vi "User_Palette.vi"(10 "Color":u32(colorbox), 11 "Palette Number (gray)":T1(ring)) -> (3 "Color Palette":cluster{"Red":u8, "Green":u8, "Blue":u8}[](array[cluster]))   [LabVIEW 2013]
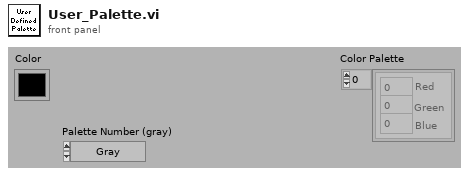
[diagram p1: front panel]
types:
  T1 = enum32{"Gray", "Binary", "Gradient", "Rainbow", "Temperature", "User Defined"}
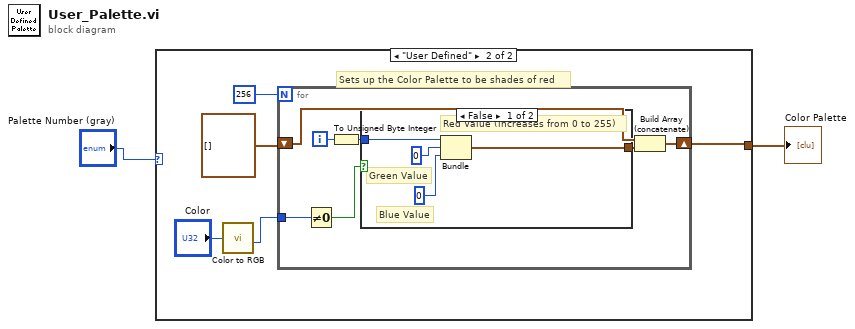
[diagram p0: block diagram]
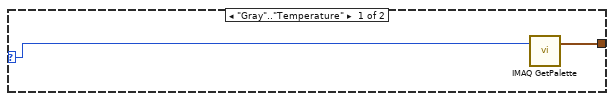
[diagram p2: hidden frame]
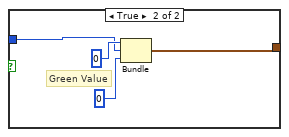
[diagram p3: hidden frame]
diagram:
  n1 = case shown="\"User Defined\"" "Palette Number (gray)" {
    selector: "Palette Number (gray)" -> [w3 _]
    tunnel: [w4 w7] -> w2
    frame "Gray".."Temperature" {
      n2 = call "IMAQ GetPalette"("Palette Number (gray)"=w3) -> ("Color Palette"=w4:cluster{"Red":u8, "Green":u8, "Blue":u8}[])  [unwired: 4 in, 1 out]
    }
    frame "User Defined" {
      # "Sets up the Color Palette to be shades of red"
      n3 = call <vilib>:"Color to RGB.vi"("Color"="Color") -> ("G"=w5:u8)  [unwired: 3 out]
      n4 = for {
        N: 256 -> [_]
        shift-right: [w14] -> w7
        shift-left: cluster{u8, "G":u8, u8}[] [] -> [w15]
        tunnel: w5 -> [w10]
        i -> [w13]
        n5 = Not Equal To 0?(x=w10) -> (x != 0?=w11:bool)
        n6 = To Unsigned Byte Integer(number=w13) -> (unsigned 8bit integer=w12:u8)
        n7 = case shown="False" w11 {
          tunnel: [w20 w21] -> w16
          tunnel: w12 -> [w18 w22]
          frame False {
            # "Red Value (increases from 0 to 255)"
            # "Blue Value"
            # "Green Value"
            n8 = Bundle(w18, "G"=u8 0, "G"=u8 0) -> (w20:cluster{u8, "G":u8, "G":u8})  [unwired: 1 in]
          }
          frame True {
            # "Green Value"
            n9 = Bundle("G"=u8 0, w22, "G"=u8 0) -> (w21:cluster{"G":u8, u8, "G":u8})  [unwired: 1 in]
          }
        }
        n10 = Build Array (concatenate)(w15, w16) -> (w14:cluster{"G":u8, "G":u8, "G":u8}[])
      }
    }
  }
  "Color Palette" <- w2
